vi "CreateByID.vi"(8 "error in (no error)":errorcluster, 10 "GaugeID":string) -> (0 "error out":errorcluster, 2 "IGauge":refnum<class "IGauge.lvclass">, 3 "GaugeFactory out":refnum<class "GaugeFactory.lvclass">)   [LabVIEW 2016, in "GaugeFactory.lvclass"]
uses:
  GaugeFactory.lvclass
  Interfaces/IGauge/IGauge.lvclass
  <vilib>/Utility/config.llb/Read Key (String).vi
  <vilib>/Utility/config.llb/NI_LVConfig.lvlib
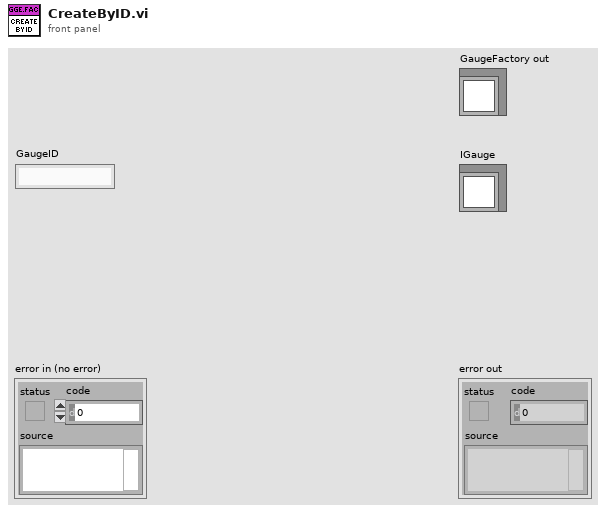
[diagram p1: front panel]
types:
  T1 = typedef "NI_LVConfig.lvlib/Config Data RefNum.ctl" = refnum<k1>
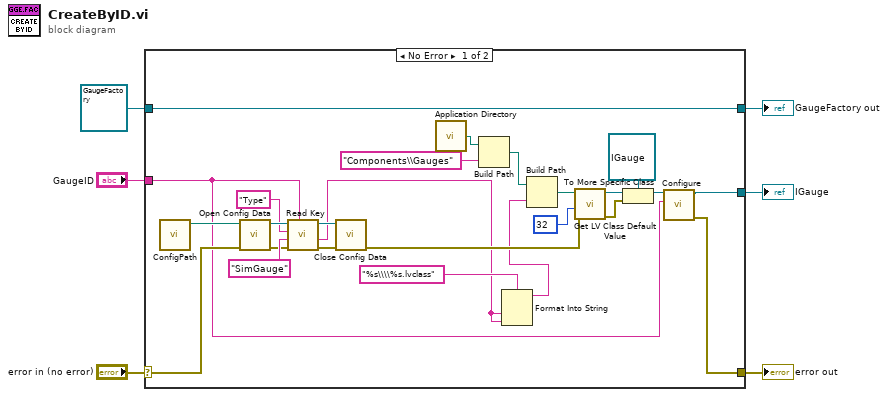
[diagram p0: block diagram]
diagram:
  n1 = case shown="No Error" "error in (no error)" {
    selector: "error in (no error)" -> [w16 w33]
    tunnel: [w7 w33] -> w5
    tunnel: [w31 w32] -> w3
    tunnel: refnum<class "GaugeFactory.lvclass"> refnum ("GaugeFactory in") -> [w31 w32]
    tunnel: "GaugeID" -> [w8 _]
    tunnel: [w9 _] -> w1
    frame No Error {
      n2 = call "ConfigPath.vi"() -> ("ConfigPath"=w23:path)  [unwired: 11 in]
      n3 = call <vilib>:"Open Config Data.vi"("error in (no error)"=w16, "configuration file path"=w23) -> ("error out"=w19:errorcluster, "refnum"=w22:T1)  [unwired: 7 in, 1 out]
      n4 = call-poly <vilib>:"Read Key.vi"("section"=w8, "error in (no error)"=w19, "default value"="SimGauge" ("key"), "key"="Type", "refnum"=w22) -> ("error out"=w17:errorcluster, "value"=w13:string, "refnum out"=w18:T1)  [unwired: 3 in, 1 out]
      n5 = call <vilib>:"Close Config Data.vi"("error in (no error)"=w17, "refnum"=w18) -> ("error out"=w15:errorcluster)  [unwired: 8 in, 1 out]
      n6 = call <vilib>:"Application Directory.vi"() -> ("Application Directory"=w30:path)
      n7 = Build Path(base path=w30, name or relative path="Components\\Gauges") -> (appended path=w25:path)
      n8 = Format Into String(format string="%s\\\\%s.lvclass", w13, w13) -> (resulting string=w12:string)  [unwired: 2 in, 1 out]
      n9 = Build Path(base path=w25, name or relative path=w12) -> (appended path=w26:path)
      n10 = call <vilib>:"Get LV Class Default Value.vi"("error in (no error)"=w15, "options"=u32 32, "class path"=w26) -> ("error out"=w27:errorcluster, "object"=w28:refnum<class>)  [unwired: 7 in]
      n11 = To More Specific Class(target class=refnum<class "IGauge.lvclass"> refnum ("IGauge.lvlib:IGauge.lvclass"), reference=w28, error in=w27) -> (specific class reference=w10:refnum<class "IGauge.lvclass">)  [unwired: 1 out]
      n12 = call-dynamic "Configure.vi"("ID"=w8, "IGauge in"=w10) -> ("error out"=w7:errorcluster, "IGauge out"=w9:refnum<class "IGauge.lvclass">)  [unwired: 8 in]
    }
    frame Error {
    }
  }
  "error out" <- w5
  "GaugeFactory out" <- w3
  "IGauge" <- w1
